vi "getWavelength_v80AM5.vi"() -> ()   [LabVIEW 2016]
uses:
  <vilib>/Analysis/baseanly.llb/Mean (DBL).vi
  x32/CLDevIFace.dll
  <vilib>/Analysis/NI_AALBase.lvlib
panel:
  out "standard deviation":dbl format="%0.5f"
  in  "# for Stdev":i32=7
  in  "Avg":i32=1
  out "Delta MHz":dbl
  in  "Scale Factor":dbl=800.0
  out "Power (mW)":dbl format="%.9f"
  out "return type":i32
  in  "Clear Chart?":bool
  in  "Delay Time (s)":dbl=0.01
  out "XY Graph":cluster{i32[], dbl[]}(graph)
  out "error out":errorcluster
  out "output param":i32
  in  "stop":bool
  in  "OK Button":bool
  out "Wavelength":dbl format="%.9f"
  in  "CommPort":dbl=6.0 caption="Comm Port #"
  # "Super cavity FSR  6 GHz\nZerodure FSR  750 MHz"
  # "1 pm = 200 MHz @1212nm\n1 pm = 800 MHz @606 nm"
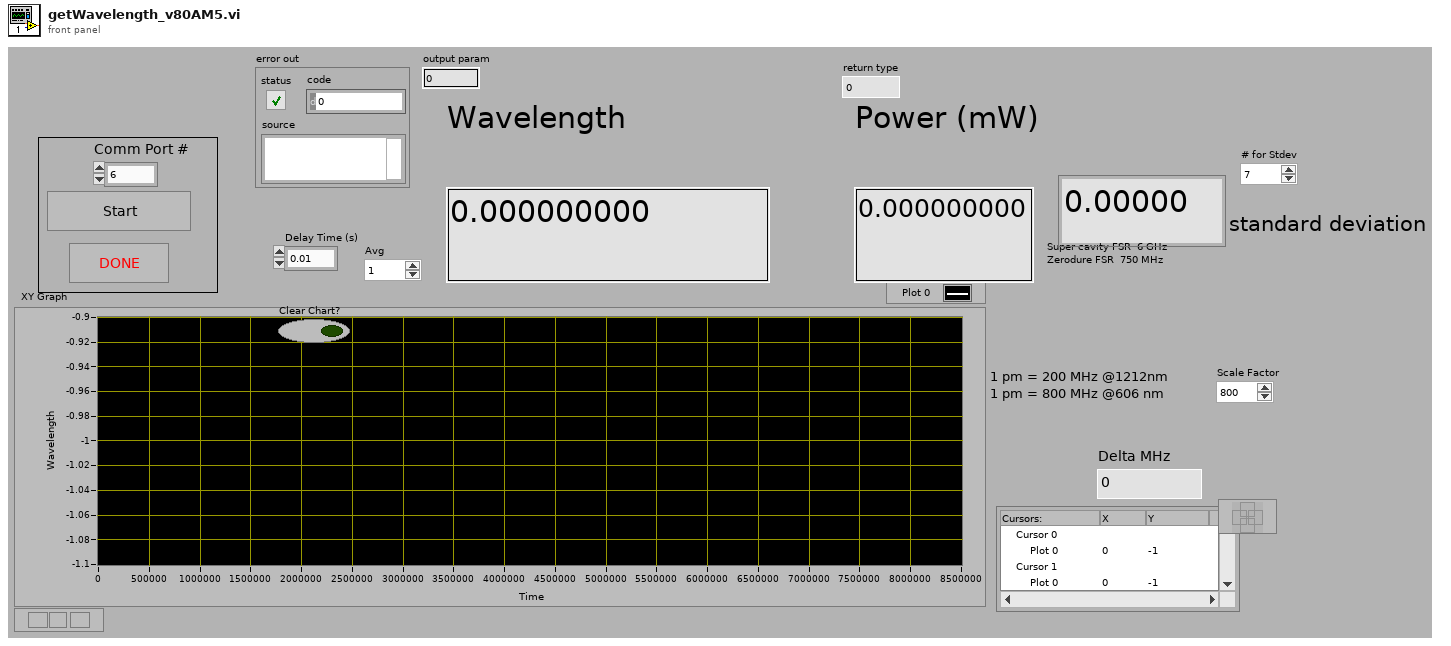
[diagram p1: front panel]
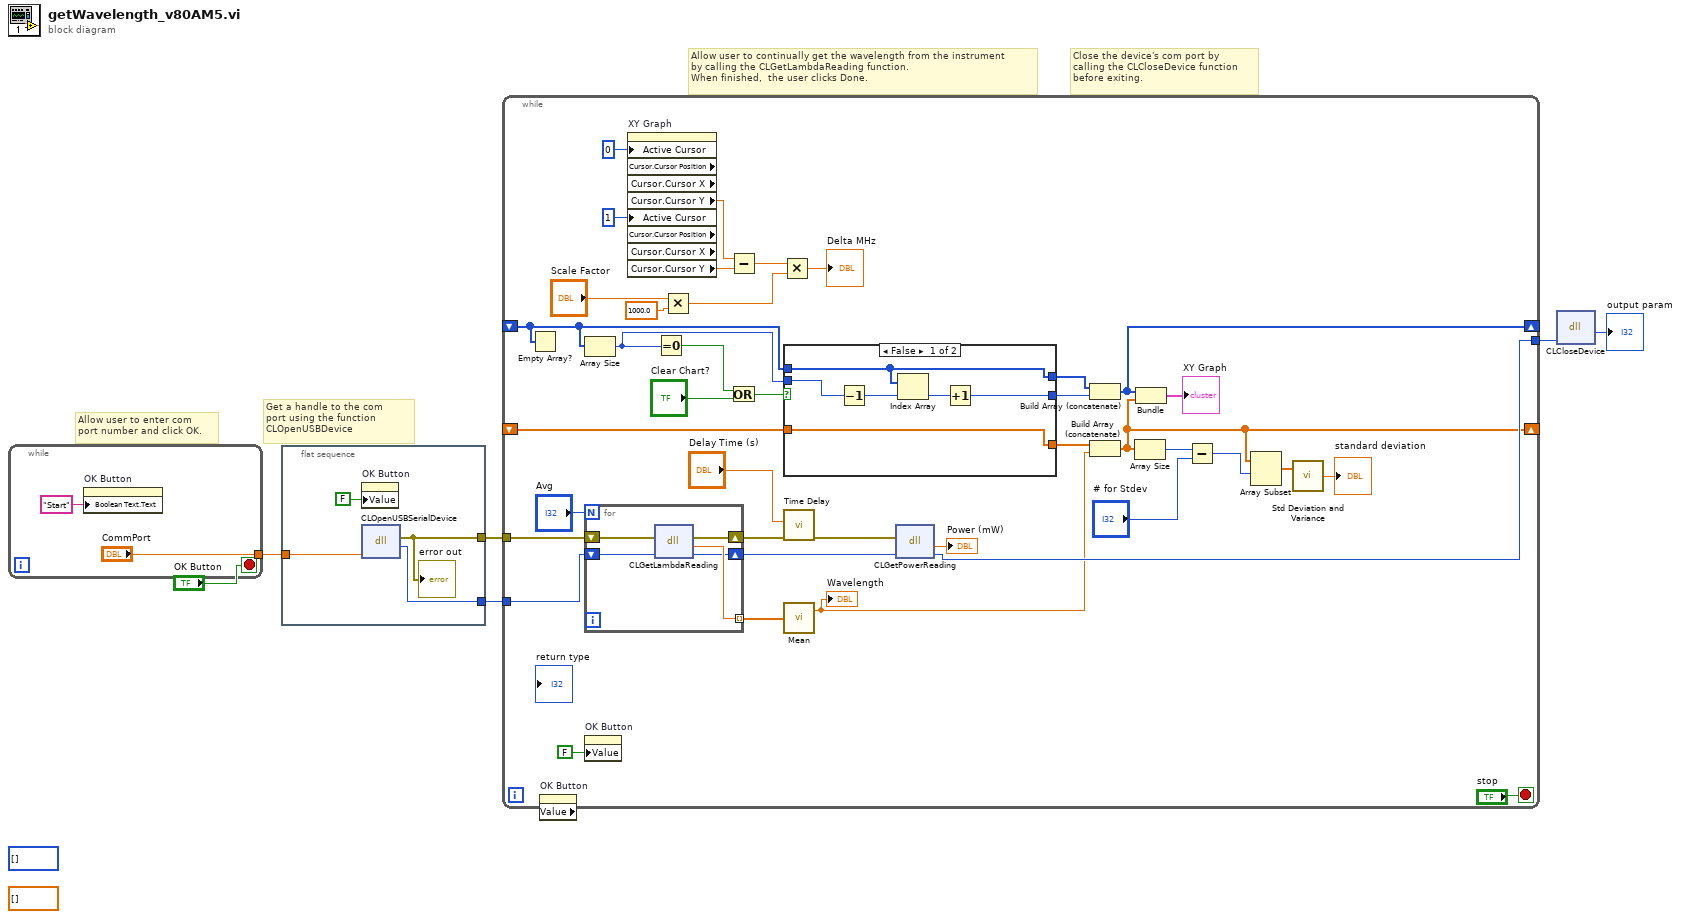
[diagram p0: block diagram]
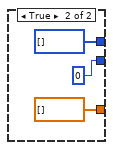
[diagram p2: hidden frame]
diagram:
  (unwired) i32[] []
  (unwired) dbl[] []
  # "Close the device's com port by\ncalling the CLCloseDevice function\nbefore exiting."
  # "Allow user to continually get the wavelength from the instrument\nby calling the CLGetLambdaReading function.  \nWhen finished,  the user clicks Done."
  # "Get a handle to the com\nport using the function CLOpenUSBDevice"
  # "Allow user to enter com \nport number and click OK."
  n1 = while {
    tunnel: ["CommPort"] -> w5
    stop <- "OK Button" stop-if-true
    n2 = property on="OK Button" class="Bool (strict)"("Boolean Text.Text"="Start") -> ()  [unwired: 2 in, 2 out]
  }
  n3 = flat-sequence {
    tunnel: w5 -> [w12]
    tunnel: [w11] -> w4
    tunnel: [w9] -> w1
    frame #0 {
      n4 = property on="OK Button" class="Bool (strict)"("Value"=FALSE) -> ()  [unwired: 2 in, 2 out]
      n5 = dll-call lib="C:/Users/Lab/Desktop/Bristol wavemeter 621/00424-2-00 621 customer CD/Programming Interface/x32/CLDevIface.dll" fn="CLOpenUSBSerialDevice"("commPort"=w12) -> (error out=w9:errorcluster, "return type"=w11:i32)  [unwired: 4 in, 1 out]
      "error out" <- w9
    }
  }
  n6 = while {
    tunnel: w4 -> [w51]
    tunnel: [w39] -> w3
    shift-right: [w18] -> _
    shift-left: _ -> [w43]
    shift-right: [w48] -> _
    shift-left: _ -> [w24]
    tunnel: w1 -> [w44]
    stop <- "stop" stop-if-true
    n7 = Empty Array?(array=w24) -> ()  [unwired: 1 out]
    n8 = property on="OK Button" class="Bool (strict)" props=["Value"]() -> ()  [unwired: 2 in, 3 out]
    n9 = Array Size(array=w24) -> (size(s)=w20:i32)
    n10 = for {
      N: "Avg" -> [_]
      tunnel: [w55] -> w22 mode=indexing
      shift-right: [w52] -> w40
      shift-left: w51 -> [w56]
      shift-right: [w54] -> w45
      shift-left: w44 -> [w53]
      n11 = dll-call lib="C:/Users/Lab/Desktop/Bristol wavemeter 621/00424-2-00 621 customer CD/Programming Interface/x32/CLDevIface.dll" fn="CLGetLambdaReading"(error in=w53, "devHandle"=w56) -> (error out=w54:errorcluster, "return type"=w55:dbl, "devHandle"=w52:i32)  [unwired: 2 in, 1 out]
    }
    n12 = property on="OK Button" class="Bool (strict)"("Value"=FALSE) -> ()  [unwired: 2 in, 2 out]
    n13 = property on="XY Graph" class="XYGraph (strict)" props=["Active Cursor", "Cursor", "Cursor Position", "Cursor", "Cursor X", "Cursor", "Cursor Y", "Active Cursor", "Cursor", "Cursor Position", "Cursor", "Cursor X", "Cursor", "Cursor Y"]("Active Cursor"=u32 0, "Active Cursor"=u32 1) -> ("Cursor.Cursor Y"=w35:dbl, "Cursor.Cursor Y"=w36:dbl)  [unwired: 2 in, 6 out]
    n14 = Equal To 0?(x=w20) -> (x = 0?=w29:bool)
    n15 = Multiply(x="Scale Factor", y=1000.0) -> (x*y=w30:dbl)
    n16 = Subtract(x=w35, y=w36) -> (x-y=w37:dbl)
    n17 = Or(x=w29, y="Clear Chart?") -> (x .or. y?=w27:bool)
    n18 = Multiply(x=w37, y=w30) -> (x*y=→"Delta MHz":dbl)
    n19 = case shown="False" w27 {
      tunnel: w43 -> [w62 _]
      tunnel: w24 -> [w61 _]
      tunnel: [w61 i32[] []] -> w25
      tunnel: [w62 dbl[] []] -> w26
      tunnel: w20 -> [w58 _]
      tunnel: [w59 0] -> w19
      frame False {
        n20 = Decrement(x=w58) -> (x-1=w57:i32)
        n21 = Index Array(array=w61, index=w57) -> (element=w60:i32)
        n22 = Increment(x=w60) -> (x+1=w59:i32)
      }
      frame True {
      }
    }
    n23 = call "Time Delay"("error in (no error)"=w45, "Delay Time (s)"="Delay Time (s)") -> ("error out"=w42:errorcluster)  [unwired: 9 in]
    n24 = call-poly <vilib>:"Mean.vi"("X"=w22) -> ("mean"=w21:dbl)  [unwired: 1 out]
    "Wavelength" <- w21
    n25 = dll-call lib="C:/Users/Lab/Desktop/Bristol wavemeter 621/00424-2-00 621 customer CD/Programming Interface/x32/CLDevIface.dll" fn="CLGetPowerReading"(error in=w42, "devHandle"=w40) -> ("return type"=→"Power (mW)":dbl, "devHandle"=w39:i32)  [unwired: 2 in, 2 out]
    n26 = Build Array (concatenate)(w25, w19) -> (w48:i32[])
    n27 = Build Array (concatenate)(w26, w21) -> (w18:dbl[])
    n28 = Array Size(array=w18) -> (size(s)=w17:i32)
    n29 = Bundle(w48, w18) -> (→"XY Graph":cluster{i32[], dbl[]})  [unwired: 1 in]
    n30 = Subtract(x=w17, y="# for Stdev") -> (x-y=w15:i32)
    n31 = Array Subset(array=w18, index=w15) -> (w14:dbl[])  [unwired: 1 in]
    n32 = call <vilib>:"Std Deviation and Variance.vi"("X"=w14) -> ("standard deviation"=→"standard deviation":dbl)  [unwired: 1 in, 2 out]
  }
  n33 = dll-call lib="C:/Users/Lab/Desktop/Bristol wavemeter 621/00424-2-00 621 customer CD/Programming Interface/x32/CLDevIface.dll" fn="CLCloseDevice"("commPort"=w3) -> ("return type"=→"output param":i32)  [unwired: 4 in, 2 out]
